vi "(SubVI)_Biuld_labels_for2DPSF.vi"(1 "Randomized Array in 2nd Dimension":dbl[](array[numeric]), 2 "Num of Stim sites":i32, 3 "Imp tab Label 3":string, 4 "Randomized Index":i32) -> (0 "concatenated string":string)   [LabVIEW 2012]
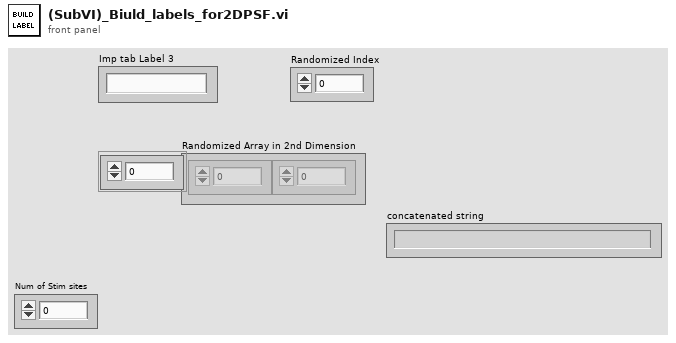
[diagram p1: front panel]
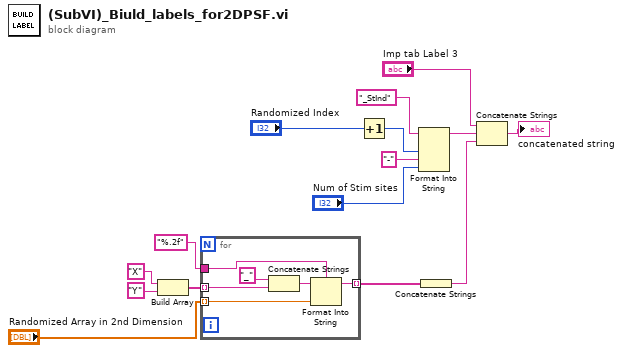
[diagram p0: block diagram]
diagram:
  n1 = Build Array("X", "Y" ("element")) -> (w11:string[])
  n2 = for {
    tunnel: "Randomized Array in 2nd Dimension" -> [w19] mode=indexing
    tunnel: [w20] -> w14 mode=indexing
    tunnel: w11 -> [w17] mode=indexing
    tunnel: "%.2f" ("format string") -> [w16]
    n3 = Concatenate Strings("_" ("string"), w17) -> (w21:string)
    n4 = Format Into String(format string=w16, initial string=w21, w19) -> (resulting string=w20:string)  [unwired: 1 in, 1 out]
  }
  n5 = Increment(x="Randomized Index") -> (x+1=w5:i32)
  n6 = Format Into String(initial string="_StInd", w5, "-" ("initial string"), "Num of Stim sites") -> (resulting string=w3:string)  [unwired: 2 in, 1 out]
  n7 = Concatenate Strings(w14) -> (w4:string)
  n8 = Concatenate Strings("Imp tab Label 3", w3, w4) -> (→"concatenated string":string)
